vi "dll_calArea.vi"(8 "error in (no error)":errorcluster, 11 "p_box":i32) -> (0 "error out":errorcluster, 2 "area":dbl, 3 "p_box":i32)   [LabVIEW 2020, in "box.lvlib"]
uses:
  box.lvlib
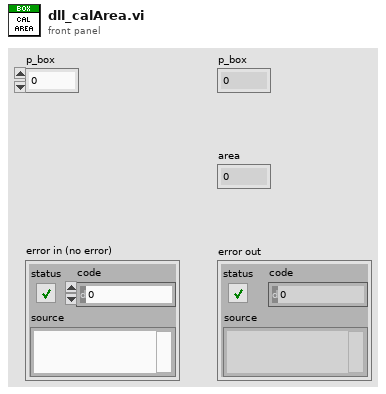
[diagram p1: front panel]
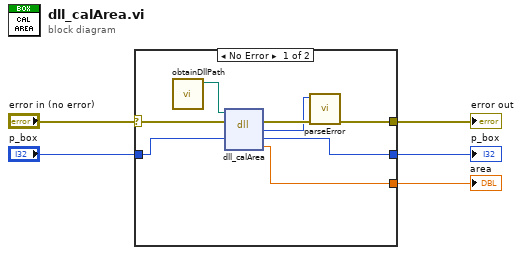
[diagram p0: block diagram]
diagram:
  n1 = case shown="No Error" "error in (no error)" {
    selector: "error in (no error)" -> [w13 w14]
    tunnel: "p_box" -> [w12 w15]
    tunnel: [w8 w14] -> w2
    tunnel: [w10 w15] -> w3
    tunnel: [w9 _] -> w1
    frame No Error {
      n2 = call "obtainDllPath.vi"() -> ("box.dll path"=w6:path)  [unwired: 11 in]
      n3 = dll-call lib="box.dll" fn="dll_calArea"(path in=w6, error in=w13, "p_box"=w12) -> (error out=w11:errorcluster, "return type"=w7:i32, "p_box"=w10:i32, "area"=w9:dbl)  [unwired: 2 in, 1 out]
      n4 = call "parseError.vi"("error in (no error)"=w11, "status code"=w7) -> ("error out"=w8:errorcluster)  [unwired: 9 in]
    }
    frame Error {
    }
  }
  "p_box" <- w3
  "error out" <- w2
  "area" <- w1
